vi "Log_Programm_Ablauf.vi"(8 "Fehler in":errorcluster, 10 "Zustand":T1, 11 "Cluster in":T2={"Initialisierung"={"Online?"=FALSE, "Grundpfad"=path "", "Kamera Oben"="", "IP-Adresse Flüssiglinse"="", "Flüssiglinse"=refnum, "Kamera Unten"="", "IP-Adresse SPS"="", "SPS-Verbindung"={"TCP Connection Ref"=refnum, "IP address"="", "timeout ms"=5000, "Connected?"=FALSE, "PLC Type"=enum."S7 1200", "Rack S7 400"=0, "Slot S7 400"=0, "PDU Size"=0, "connection semaphore"=refnum}, "IP-Adresse Lichtgitter"="", "Lichtgitter"=refnum, "Bilder Oben"=[], "Bild Unten"=refnum}, "Einstellungen"={"i. O. Bilder speichern"=FALSE, "Ausgewähltes Offline-Datum"="", "Ausgewähltes Offline-Teil"="", "Speicherpfad Bilder"=path ""}, "Artikeldaten"={"Artikelnummer"="", "Fertigungsauftrag"="", "Belichtungszeit Referenzmarken"=0.0, "Fokus Referenzmarken"=0.0, "Belichtungszeit ISO"=0.0, "Fokus ISO"=0.0, "Belichtungszeit Kontakte"=0.0, "Fokus Kontakte"=0.0, "Belichtungszeit Unten"=0.0, "Kontaktanzahl"=0, "Kontaktpositionen"=[], "Aktueller Kontakt"=0}, "Kamera Oben"={"Position Kontakt"={"x"=0.0, "y"=0.0}, "Prüfung Oben i. O."=FALSE}, "Kamera Unten"={"Prüfung Unten i. O."=FALSE}, "Messung Lichtgitter"={"Kontakt & WT in Lichtgitter?"=FALSE, "Aktuelle Messwerte"=[], "Offset"={"x"=0.0, "y"=0.0}}, "Statistik"={"Statistiken"=[]}}) -> (0 "Fehler out":errorcluster, 3 "Cluster out":T2={"Initialisierung"={"Online?"=FALSE, "Grundpfad"=path "", "Kamera Oben"="", "IP-Adresse Flüssiglinse"="", "Flüssiglinse"=refnum, "Kamera Unten"="", "IP-Adresse SPS"="", "SPS-Verbindung"={"TCP Connection Ref"=refnum, "IP address"="", "timeout ms"=5000, "Connected?"=FALSE, "PLC Type"=enum."S7 1200", "Rack S7 400"=0, "Slot S7 400"=0, "PDU Size"=0, "connection semaphore"=refnum}, "IP-Adresse Lichtgitter"="", "Lichtgitter"=refnum, "Bilder Oben"=[], "Bild Unten"=refnum}, "Einstellungen"={"i. O. Bilder speichern"=FALSE, "Ausgewähltes Offline-Datum"="", "Ausgewähltes Offline-Teil"="", "Speicherpfad Bilder"=path ""}, "Artikeldaten"={"Artikelnummer"="", "Fertigungsauftrag"="", "Belichtungszeit Referenzmarken"=0.0, "Fokus Referenzmarken"=0.0, "Belichtungszeit ISO"=0.0, "Fokus ISO"=0.0, "Belichtungszeit Kontakte"=0.0, "Fokus Kontakte"=0.0, "Belichtungszeit Unten"=0.0, "Kontaktanzahl"=0, "Kontaktpositionen"=[], "Aktueller Kontakt"=0}, "Kamera Oben"={"Position Kontakt"={"x"=0.0, "y"=0.0}, "Prüfung Oben i. O."=FALSE}, "Kamera Unten"={"Prüfung Unten i. O."=FALSE}, "Messung Lichtgitter"={"Kontakt & WT in Lichtgitter?"=FALSE, "Aktuelle Messwerte"=[], "Offset"={"x"=0.0, "y"=0.0}}, "Statistik"={"Statistiken"=[]}})   [LabVIEW 2024]
uses:
  Typdefinitionen/Cluster.ctl
  <vilib>/userDefined/High Color/IMAQdx.ctl
  <vilib>/DATA AHEAD/SP7/typedefs/S7 Connection.ctl
  <vilib>/DATA AHEAD/SP7/typedefs/PLC Type.ctl
  <vilib>/vision/Image Controls.llb/IMAQ Image.ctl
  Typdefinitionen/Statistik.ctl
  Typdefinitionen/Zustand.ctl
  <vilib>/Utility/file.llb/Write Delimited Spreadsheet (string).vi
  <vilib>/DATA AHEAD/SP7/SP7.lvlib
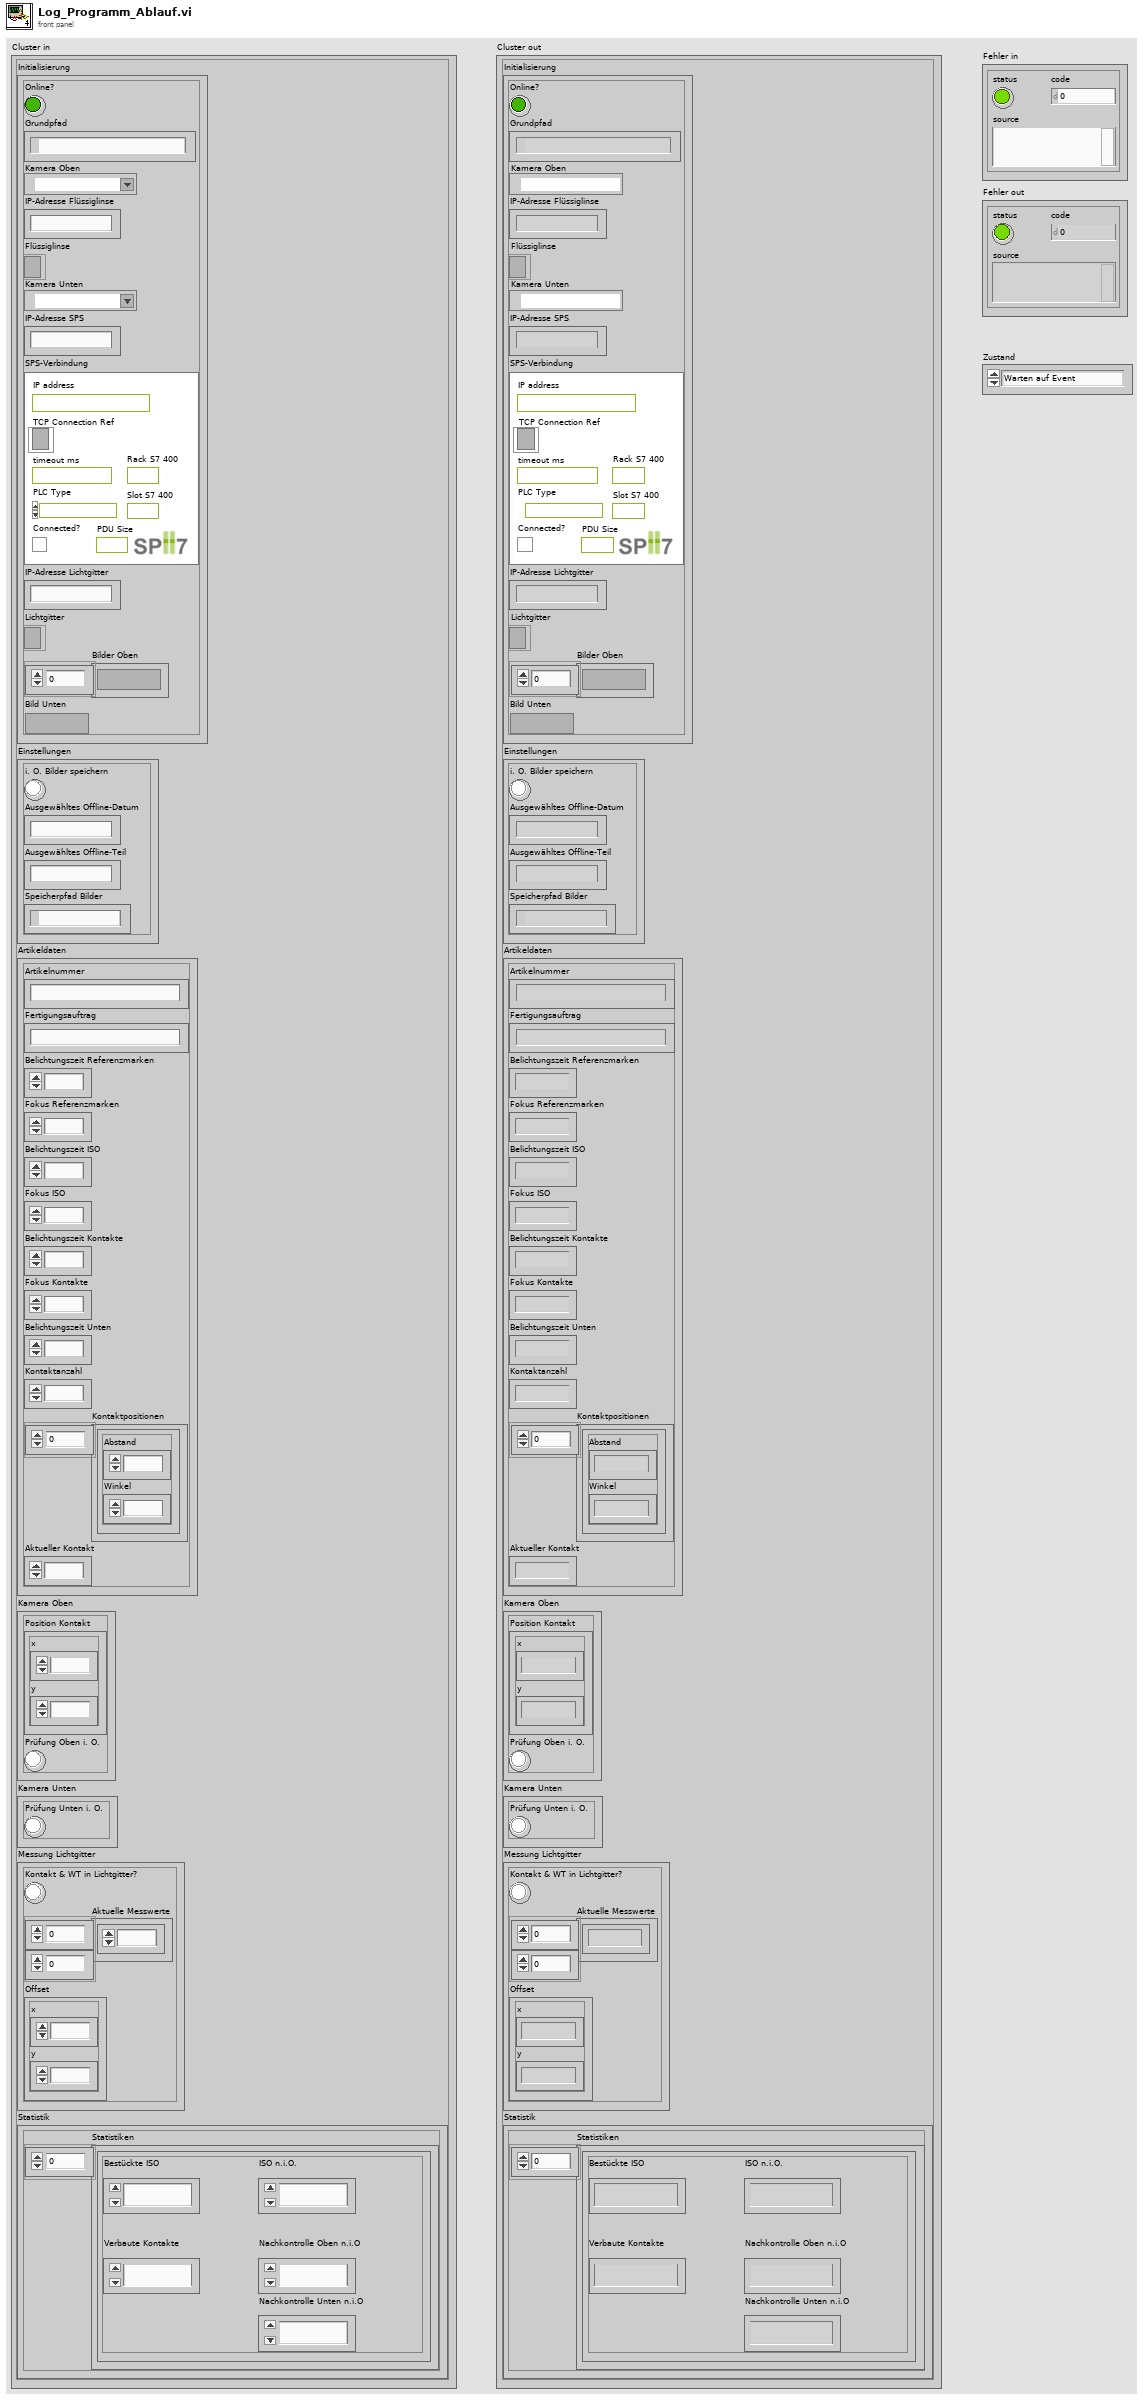
[diagram p1: front panel]
types:
  T1 = typedef "Zustand.ctl" = enum16{"Warten auf Event", "Artikeldaten laden", "Init Prüfung Oben", "Bildaufnahme Oben", "Auswertung Oben", "Init Vermessung Lichtgitter", "Messwertaufnahme Lichtgitter", "Auswertung Lichtgitter", "Init Prüfung Unten", "Bildaufnahme Unten", "Auswertung Unten", "ISO & Referenzbohrungen speichern", "Nachkontrolle speichern"}
  T2 = typedef "Cluster.ctl" = cluster{"Initialisierung":cluster{"Online?":bool, "Grundpfad":path, "Kamera Oben":T3, "IP-Adresse Flüssiglinse":string, "Flüssiglinse":refnum<k5>, "Kamera Unten":T3, "IP-Adresse SPS":string, "SPS-Verbindung":T4, "IP-Adresse Lichtgitter":string, "Lichtgitter":refnum<k5>, "Bilder Oben":T7[], "Bild Unten":T7}, "Einstellungen":cluster{"i. O. Bilder speichern":bool, "Ausgewähltes Offline-Datum":string, "Ausgewähltes Offline-Teil":string, "Speicherpfad Bilder":path}, "Artikeldaten":cluster{"Artikelnummer":string, "Fertigungsauftrag":string, "Belichtungszeit Referenzmarken":dbl, "Fokus Referenzmarken":dbl, "Belichtungszeit ISO":dbl, "Fokus ISO":dbl, "Belichtungszeit Kontakte":dbl, "Fokus Kontakte":dbl, "Belichtungszeit Unten":dbl, "Kontaktanzahl":u32, "Kontaktpositionen":cluster{"Abstand":dbl, "Winkel":dbl}[], "Aktueller Kontakt":u32}, "Kamera Oben":cluster{"Position Kontakt":cluster{"x":dbl, "y":dbl}, "Prüfung Oben i. O.":bool}, "Kamera Unten":cluster{"Prüfung Unten i. O.":bool}, "Messung Lichtgitter":cluster{"Kontakt & WT in Lichtgitter?":bool, "Aktuelle Messwerte":dbl[][], "Offset":cluster{"x":dbl, "y":dbl}}, "Statistik":cluster{"Statistiken":T8[]}}
  T3 = typedef "IMAQdx.ctl" = refnum<k21>
  T4 = typedef "SP7.lvlib/S7 Connection.ctl" = cluster{"TCP Connection Ref":refnum<k5>, "IP address":string, "timeout ms":i32, "Connected?":bool, "PLC Type":T5, "Rack S7 400":u8, "Slot S7 400":u8, "PDU Size":u16, "connection semaphore":T6}
  T5 = typedef "SP7.lvlib/PLC Type.ctl" = enum16{"S7 200", "S7 300/400", "S7 1200", "S7 1500", "LOGO!8"}
  T6 = typedef "Semaphore RefNum" = refnum<k1>
  T7 = typedef "IMAQ Image.ctl" = refnum<image>
  T8 = typedef "Statistik.ctl" = cluster{"Bestückte ISO":u32, "Verbaute Kontakte":u32, "ISO n.i.O.":u32, "Nachkontrolle Oben n.i.O":u32, "Nachkontrolle Unten n.i.O":u32}
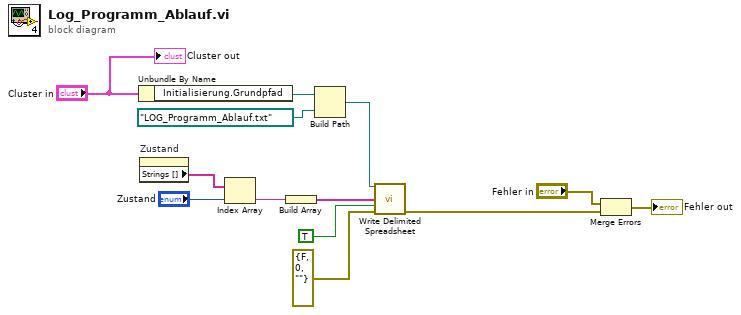
[diagram p0: block diagram]
diagram:
  n1 = Unbundle By Name("Cluster in") -> ("Initialisierung.Grundpfad"=w11:path)
  n2 = property on="Zustand" class="Enum (strict)"() -> ("Strings []"=w7:string[])  [unwired: 2 in, 2 out]
  n3 = Index Array(array=w7, index="Zustand") -> (element=w5:string)
  n4 = Build Array(w5) -> (w4:string[])
  n5 = Build Path(base path=w11, name or relative path=path "LOG_Programm_Ablauf.txt") -> (appended path=w9:path)
  n6 = call-poly <vilib>:"Write Delimited Spreadsheet.vi"("file path (dialog if empty)"=w9, "1D data"=w4, "append to file? (new file:F)"=TRUE, "error in (no error)"=errorcluster {"status"=FALSE, "code"=0, "source"=""}) -> ("error out"=w2:errorcluster)  [unwired: 10 in, 1 out]
  n7 = Merge Errors("Fehler in", w2) -> (→"Fehler out":errorcluster)
  "Cluster out" <- "Cluster in"
